vi "GEA2 Serial Send ACK.vi"(8 "error in (no error)":errorcluster, 10 "CRC":bool, 11 "VISA Refnum in":refnum<visa-resource-name>) -> (0 "error out":errorcluster)   [LabVIEW 2014]
uses:
  Type Definitions/GEA2 Serial Dryer Error Enumeration.ctl
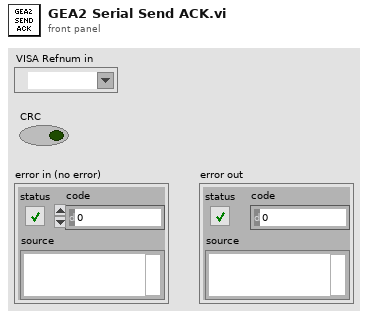
[diagram p1: front panel]
types:
  T1 = typedef "GEA2 Serial Dryer Error Enumeration.ctl" = enum16{"No Error", "GEA2 Send ACK Mismatch", "GEA2 STX", "GEA2 ETX", "GEA2 CRC Mismatch", "GEA2 ReadACK", "RTD In Range Error", "Fail Mean Tank Temp", "No Flow Config Data Found", "Failed Flow During Purge", "Temp During Purge", "Confirm IF Stop Fail", "Init Draw: TC_1 Out of Range", "Flow = 0 During Draw after 20s"}
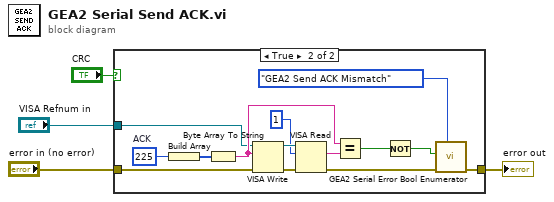
[diagram p0: block diagram]
diagram:
  n1 = case shown="True" "CRC" {
    tunnel: "error in (no error)" -> [w5 w19]
    tunnel: "VISA Refnum in" -> [_ w13]
    tunnel: [w5 w12] -> w3
    frame False {
    }
    frame True {
      w14 = u8 225  # ACK
      n2 = Build Array(w14) -> (w17:u8[])
      n3 = Byte Array To String(unsigned byte array=w17) -> (string=w16:string)
      n4 = VISA Write(VISA resource name=w13, write buffer=w16, error in (no error)=w19) -> (VISA resource name out=w18:refnum<visa-resource-name>, error out=w15:errorcluster)  [unwired: 1 out]
      n5 = VISA Read(VISA resource name=w18, byte count=u32 1, error in (no error)=w15) -> (read buffer=w9:string, error out=w10:errorcluster)  [unwired: 2 out]
      n6 = Equal?(x=w16, y=w9) -> (x = y?=w7:bool)
      n7 = Not(x=w7) -> (.not. x?=w6:bool)
      n8 = call "GEA2 Serial Error Bool Enumerator.vi"("Error Enum"=GEA2_Serial_Dryer_Error_Enumeration."GEA2 Send ACK Mismatch", "Error In"=w10, "Error?"=w6) -> ("Error Out"=w12:errorcluster)  [unwired: 6 in]
    }
  }
  "error out" <- w3
